vi "Measurement Parser.vi"(7 "Waveform Graph":dynamicdata(graph), 8 "error in (no error)":errorcluster, 9 "Generic Card in":refnum<class "Generic Card.lvclass">, 10 "Data Array":dbl[](array[numeric]), 11 "Tektronix DMM4020 in":refnum<class "Tektronix DMM4020.lvclass">) -> (0 "error out":errorcluster, 3 "Tektronix DMM4020 out":refnum<class "Tektronix DMM4020.lvclass">)   [LabVIEW 2016, in "Generic Digital Multi Meter.lvlib" / "Tektronix DMM4020.lvlib" / "Tektronix DMM4020.lvclass"]
uses:
  Tektronix DMM4020.lvclass
  Generic Instrument/Generic Card/Generic Card.lvclass
  Generic Digita Multi Meter/Generic Digital Multi Meter.lvclass
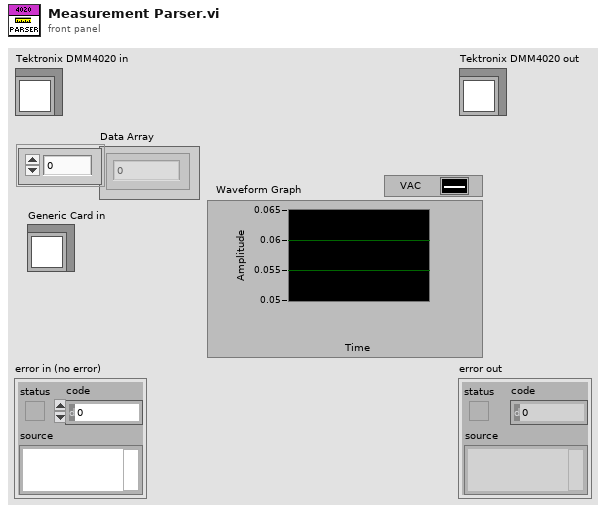
[diagram p1: front panel]
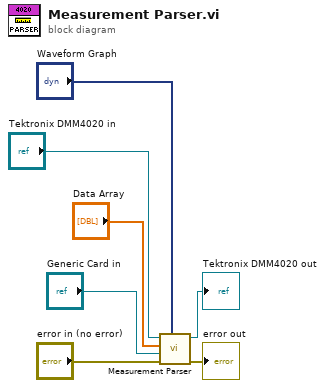
[diagram p0: block diagram]
diagram:
  n1 = call-parent "Measurement Parser.vi"("Waveform Graph"="Waveform Graph", "error in (no error)"="error in (no error)", "Generic Card in"="Generic Card in", "Data Array"="Data Array", "Generic Digital Multi Meter in"="Tektronix DMM4020 in") -> ("error out"=→"error out":errorcluster, "Generic Digital Multi Meter out"=→"Tektronix DMM4020 out":refnum<class "Tektronix DMM4020.lvclass">)  [unwired: 5 in]
